vi "eeprom-recode.vi"(0 "PWM":T1, 2 "Rotulo izquierdo:":string, 3 "Rotulo derecho:":string, 4 "Cant Med:":u8, 5 "Medición Ampliada:":u8, 6 "DIG_16":T2(array[cluster]), 7 "DIG_8":T2(array[cluster]), 8 "Ana 32":T3(array[cluster]), 9 "Ana 16":T3(array[cluster])) -> (1 "Recoded eeprom":string)   [LabVIEW 2010]
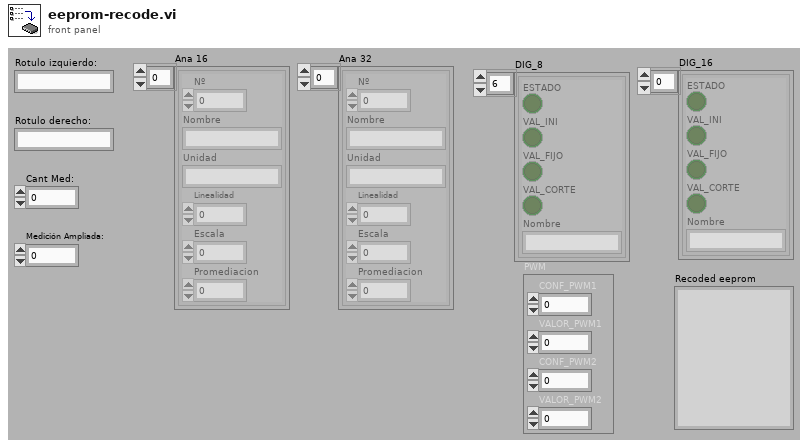
[diagram p1: front panel]
types:
  T1 = cluster{"CONF_PWM1":u8, "VALOR_PWM1":u8, "CONF_PWM2":u8, "VALOR_PWM2":u8}
  T2 = cluster{"ESTADO":bool, "VAL_INI":bool, "VAL_FIJO":bool, "VAL_CORTE":bool, "Nombre":string}[]
  T3 = cluster{"Nº":i32, "Nombre":string, "Unidad":string, "Linealidad":u8, "Escala":u8, "Promediacion":u8}[]
  T4 = cluster{"[0]":cluster{"Nº":i32, "Nombre":string, "Unidad":string, "Linealidad":u8, "Escala":u8, "Promediacion":u8}}
  T5 = cluster{"Nº":i32, "Nombre":string, "Unidad":string, "Linealidad":u8, "Escala":u8, "Promediacion":u8}
  T6 = cluster{"[0]":cluster{"ESTADO":bool, "VAL_INI":bool, "VAL_FIJO":bool, "VAL_CORTE":bool, "Nombre":string}}
  T7 = cluster{"ESTADO":bool, "VAL_INI":bool, "VAL_FIJO":bool, "VAL_CORTE":bool, "Nombre":string}
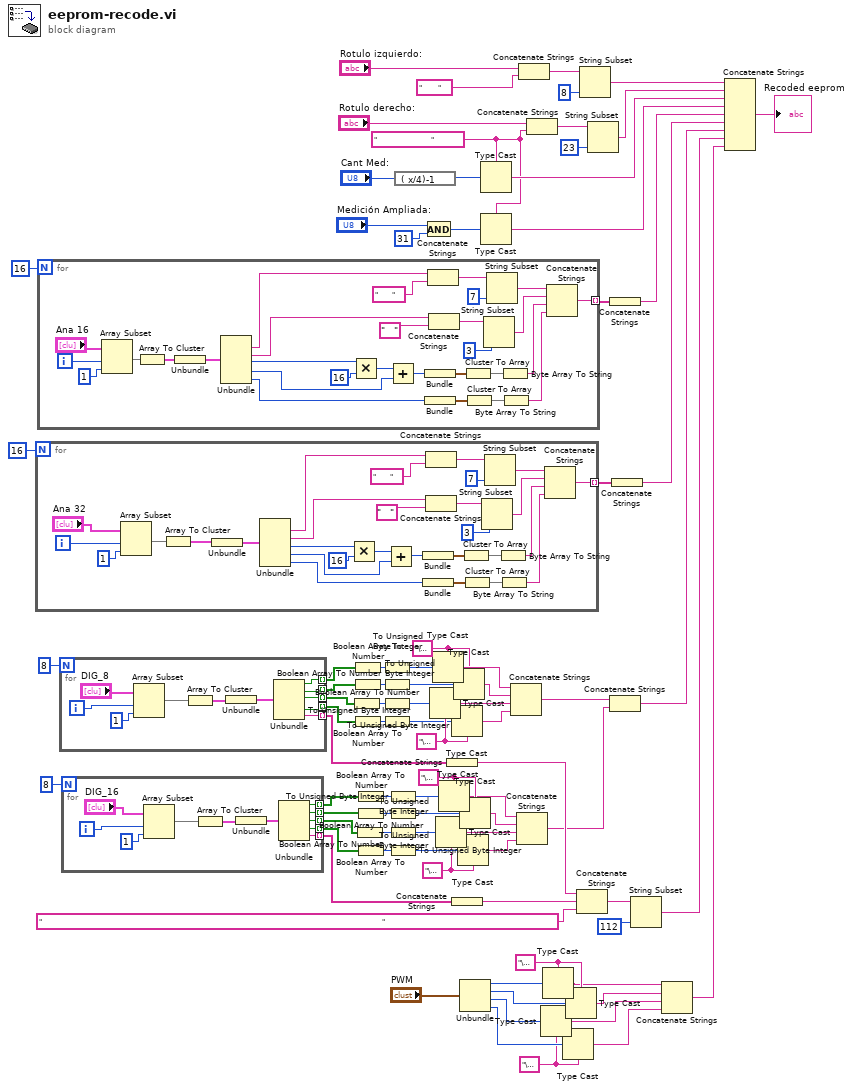
[diagram p0: block diagram]
diagram:
  w28 = "\u0000"
  w27 = "\u0000"
  w50 = "\u0000"
  w51 = "\u0000"
  w62 = "\u0000"
  w63 = "\u0000"
  w4 = "                           " ("string")
  n1 = for {
    N: 16 -> [_]
    tunnel: [w87] -> w10 mode=indexing
    i -> [w88]
    n2 = Array Subset(array="Ana 32", index=w88, length=1) -> (w113:T3)
    n3 = Array To Cluster(array=w113) -> (cluster=w112:T4)
    n4 = Unbundle(w112) -> ("[0]"=w111:T5)
    n5 = Unbundle(w111) -> ("Nombre"=w93:string, "Unidad"=w92:string, "Linealidad"=w91:u8, "Escala"=w90:u8, "Promediacion"=w89:u8)  [unwired: 1 out]
    n6 = Multiply(x=w91, y=u8 16) -> (x*y=w103:u8)
    n7 = Add(x=w103, y=w90) -> (x+y=w104:u8)
    n8 = Bundle(w104) -> (w105:cluster{u8})  [unwired: 1 in]
    n9 = Bundle("Promediacion"=w89) -> (w109:cluster{"Promediacion":u8})  [unwired: 1 in]
    n10 = Concatenate Strings(w93, "       " ("string")) -> (w95:string)
    n11 = Concatenate Strings(w92, "   " ("string")) -> (w98:string)
    n12 = Cluster To Array(cluster=w105) -> (array=w106:u8[])
    n13 = Cluster To Array(cluster=w109) -> (array=w108:u8[])
    n14 = String Subset(string=w98, length (rest)=3 ("length (rest)")) -> (substring=w100:string)  [unwired: 1 out]
    n15 = String Subset(string=w95, length (rest)=7 ("length (rest)")) -> (substring=w101:string)  [unwired: 1 out]
    n16 = Byte Array To String(unsigned byte array=w106) -> (string=w107:string)
    n17 = Byte Array To String(unsigned byte array=w108) -> (string=w110:string)
    n18 = Concatenate Strings(w101, w100, w107, w110) -> (w87:string)
  }
  n19 = for {
    N: 16 -> [_]
    tunnel: [w117] -> w12 mode=indexing
    i -> [w118]
    n20 = Array Subset(array="Ana 16", index=w118, length=1) -> (w142:T3)
    n21 = Array To Cluster(array=w142) -> (cluster=w141:T4)
    n22 = Unbundle(w141) -> ("[0]"=w115:T5)
    n23 = Unbundle(w115) -> ("Nombre"=w122:string, "Unidad"=w121:string, "Linealidad"=w120:u8, "Escala"=w116:u8, "Promediacion"=w119:u8)  [unwired: 1 out]
    n24 = Multiply(x=w120, y=u8 16) -> (x*y=w132:u8)
    n25 = Add(x=w132, y=w116) -> (x+y=w133:u8)
    n26 = Bundle(w133) -> (w134:cluster{u8})  [unwired: 1 in]
    n27 = Bundle("Promediacion"=w119) -> (w138:cluster{"Promediacion":u8})  [unwired: 1 in]
    n28 = Concatenate Strings(w122, "       " ("string")) -> (w124:string)
    n29 = Concatenate Strings(w121, "   " ("string")) -> (w127:string)
    n30 = Cluster To Array(cluster=w134) -> (array=w135:u8[])
    n31 = Cluster To Array(cluster=w138) -> (array=w137:u8[])
    n32 = String Subset(string=w127, length (rest)=3 ("length (rest)")) -> (substring=w129:string)  [unwired: 1 out]
    n33 = String Subset(string=w124, length (rest)=7 ("length (rest)")) -> (substring=w130:string)  [unwired: 1 out]
    n34 = Byte Array To String(unsigned byte array=w135) -> (string=w136:string)
    n35 = Byte Array To String(unsigned byte array=w137) -> (string=w139:string)
    n36 = Concatenate Strings(w130, w129, w136, w139) -> (w117:string)
  }
  n37 = for {
    N: 8 -> [_]
    tunnel: [w148] -> w72 mode=indexing
    tunnel: [w147] -> w49 mode=indexing
    tunnel: [w146] -> w46 mode=indexing
    tunnel: [w145] -> w47 mode=indexing
    tunnel: [w144] -> w48 mode=indexing
    i -> [w152]
    n38 = Array Subset(array="DIG_8", index=w152, length=1) -> (w149:T2)
    n39 = Array To Cluster(array=w149) -> (cluster=w151:T6)
    n40 = Unbundle(w151) -> ("[0]"=w150:T7)
    n41 = Unbundle(w150) -> ("ESTADO"=w147:bool, "VAL_INI"=w144:bool, "VAL_FIJO"=w145:bool, "VAL_CORTE"=w146:bool, "Nombre"=w148:string)
  }
  n42 = for {
    N: 8 -> [_]
    tunnel: [w159] -> w71 mode=indexing
    tunnel: [w158] -> w21 mode=indexing
    tunnel: [w157] -> w20 mode=indexing
    tunnel: [w156] -> w19 mode=indexing
    tunnel: [w155] -> w18 mode=indexing
    i -> [w164]
    n43 = Array Subset(array="DIG_16", index=w164, length=1) -> (w161:T2)
    n44 = Array To Cluster(array=w161) -> (cluster=w163:T6)
    n45 = Unbundle(w163) -> ("[0]"=w162:T7)
    n46 = Unbundle(w162) -> ("ESTADO"=w158:bool, "VAL_INI"=w157:bool, "VAL_FIJO"=w156:bool, "VAL_CORTE"=w155:bool, "Nombre"=w159:string)
  }
  n47 = Boolean Array To Number(Boolean array=w47) -> (number=w42:u32)
  n48 = Boolean Array To Number(Boolean array=w49) -> (number=w44:u32)
  n49 = Boolean Array To Number(Boolean array=w48) -> (number=w43:u32)
  n50 = Boolean Array To Number(Boolean array=w46) -> (number=w41:u32)
  n51 = Boolean Array To Number(Boolean array=w19) -> (number=w31:u32)
  n52 = Boolean Array To Number(Boolean array=w21) -> (number=w29:u32)
  n53 = Boolean Array To Number(Boolean array=w20) -> (number=w30:u32)
  n54 = Boolean Array To Number(Boolean array=w18) -> (number=w32:u32)
  n55 = To Unsigned Byte Integer(number=w44) -> (unsigned 8bit integer=w37:u8)
  n56 = To Unsigned Byte Integer(number=w43) -> (unsigned 8bit integer=w38:u8)
  n57 = To Unsigned Byte Integer(number=w42) -> (unsigned 8bit integer=w39:u8)
  n58 = To Unsigned Byte Integer(number=w41) -> (unsigned 8bit integer=w40:u8)
  n59 = To Unsigned Byte Integer(number=w29) -> (unsigned 8bit integer=w36:u8)
  n60 = To Unsigned Byte Integer(number=w30) -> (unsigned 8bit integer=w35:u8)
  n61 = To Unsigned Byte Integer(number=w31) -> (unsigned 8bit integer=w34:u8)
  n62 = To Unsigned Byte Integer(number=w32) -> (unsigned 8bit integer=w33:u8)
  n63 = expression code="( x/4)-1"("Cant Med:") -> (w5:u8)
  n64 = And(x="Medición Ampliada:", y=u8 31) -> (x .and. y?=w2:u8)
  n65 = Type Cast(type=w50, x=w39) -> (*(type *) &x=w53:string)
  n66 = Type Cast(type=w51, x=w37) -> (*(type *) &x=w55:string)
  n67 = Type Cast(type=w28, x=w34) -> (*(type *) &x=w25:string)
  n68 = Type Cast(type=w27, x=w36) -> (*(type *) &x=w23:string)
  n69 = Concatenate Strings(w72) -> (w70:string)
  n70 = Type Cast(type=w50, x=w40) -> (*(type *) &x=w54:string)
  n71 = Concatenate Strings(w71) -> (w69:string)
  n72 = Type Cast(type=w51, x=w38) -> (*(type *) &x=w52:string)
  n73 = Type Cast(type=w28, x=w33) -> (*(type *) &x=w24:string)
  n74 = Type Cast(type=w27, x=w35) -> (*(type *) &x=w26:string)
  n75 = Unbundle("PWM") -> ("CONF_PWM1"=w67:u8, "VALOR_PWM1"=w66:u8, "CONF_PWM2"=w65:u8, "VALOR_PWM2"=w64:u8)
  n76 = Type Cast(type=w4, x=w5) -> (*(type *) &x=w6:string)
  n77 = Type Cast(type=w4, x=w2) -> (*(type *) &x=w7:string)
  n78 = Concatenate Strings(w55, w52, w53, w54) -> (w45:string)
  n79 = Concatenate Strings(w23, w26, w25, w24) -> (w22:string)
  n80 = Concatenate Strings("Rotulo izquierdo:", "        " ("string")) -> (w83:string)
  n81 = Concatenate Strings("Rotulo derecho:", w4) -> (w82:string)
  n82 = Type Cast(type=w62, x=w65) -> (*(type *) &x=w59:string)
  n83 = Type Cast(type=w63, x=w67) -> (*(type *) &x=w61:string)
  n84 = Type Cast(type=w62, x=w64) -> (*(type *) &x=w58:string)
  n85 = Type Cast(type=w63, x=w66) -> (*(type *) &x=w60:string)
  n86 = Concatenate Strings(w70, w69, "                                                                                                                                                                          " ("string")) -> (w56:string)
  n87 = String Subset(string=w83, length (rest)=8 ("length (rest)")) -> (substring=w17:string)  [unwired: 1 out]
  n88 = String Subset(string=w82, length (rest)=23 ("length (rest)")) -> (substring=w16:string)  [unwired: 1 out]
  n89 = Concatenate Strings(w12) -> (w11:string)
  n90 = Concatenate Strings(w45, w22) -> (w15:string)
  n91 = Concatenate Strings(w10) -> (w9:string)
  n92 = String Subset(string=w56, length (rest)=112 ("length (rest)")) -> (substring=w14:string)  [unwired: 1 in]
  n93 = Concatenate Strings(w61, w60, w59, w58) -> (w13:string)
  n94 = Concatenate Strings(w17, w16, w6, w7, w11, w9, w15, w14, w13) -> (→"Recoded eeprom":string)
